vi "Read String.vi"(8 "error in":errorcluster, 11 "String Control Reference in":refnum<vi>) -> (0 "error out":errorcluster, 1 "Value":string, 2 "Interpret As Unicode":bool, 3 "String Control Reference out":refnum<vi>)   [LabVIEW 2020, in "G-Unicode.lvlib"]
uses:
  G-Unicode.lvlib
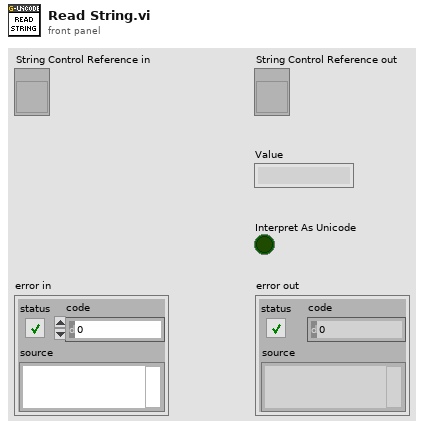
[diagram p1: front panel]
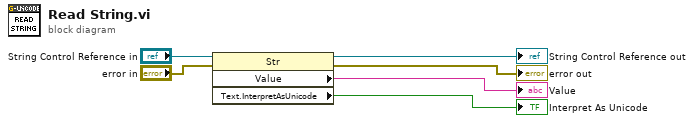
[diagram p0: block diagram]
diagram:
  n1 = property class="Str"(reference="String Control Reference in", error in="error in") -> (reference out=→"String Control Reference out":refnum<vi>, error out=→"error out":errorcluster, "Value"=→"Value":string, "Text.InterpretAsUnicode"=→"Interpret As Unicode":bool)
